vi "Dynamic Launch Nested Actor.vi"(8 "error in (no error)":errorcluster, 11 "UI ActorTop in":refnum<class "UI_Top.lvclass">) -> (0 "error out":errorcluster, 3 "UI ActorTop out":refnum<class "UI_Top.lvclass">)   [LabVIEW 2021, in "UI_Top.lvclass"]
doc: "Use Launch Nested Actor.vi to dynamic load child VI.\n2015-04-02 12:54:56\n蒋松\njiangsong@outlook.com"
uses:
  UI_Top.lvclass
  C:/Program Files (x86)/National Instruments/LabVIEW 2021/vi.lib/ActorFramework/Actor/Actor.lvclass
  C:/Program Files (x86)/National Instruments/LabVIEW 2021/user.lib/John_Lib/AbstractActorTemplate/AbstractActorTemplate/UIActorTop.lvclass
  UI_Top.lvclass/UI_Top.ctl
  <vilib>/ActorFramework/Actor/Actor.lvclass
  C:/Program Files (x86)/National Instruments/LabVIEW 2021/project/Create Actor from Template/Source_DataViewer/UI_Top/UI_Top.lvclass
  C:/Program Files (x86)/National Instruments/LabVIEW 2021/user.lib/John_Lib/Interfaces/InsertMainSubPanel/InsertMainSubPanel.lvclass
  C:/Program Files (x86)/National Instruments/LabVIEW 2021/user.lib/John_Lib/Interfaces/Windows Title/Windows Title.lvclass
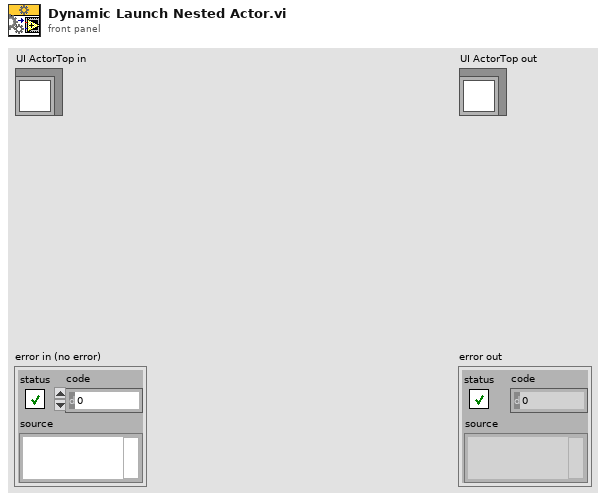
[diagram p1: front panel]
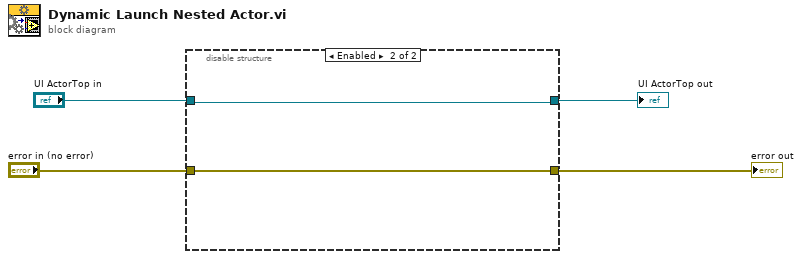
[diagram p0: block diagram]
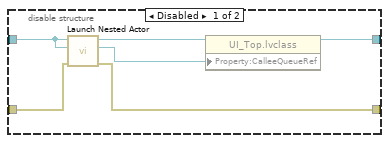
[diagram p2: hidden frame]
diagram:
  n1 = disable-structure shown="Enabled" {
    disable-tunnel: "error in (no error)" -> [w9 w11]
    disable-tunnel: [w8 w11] -> w3
    disable-tunnel: [w7 w12] -> w2
    disable-tunnel: "UI ActorTop in" -> [w5 w12]
    frame Disabled {
      n2 = call <vilib>:"Launch Nested Actor.vi"("error in (no error)"=w9, "Nested Actor"=w5, "Caller Actor in"=w5) -> ("error out"=w8:errorcluster, "Nested Actor's Enqueuer"=w6:refnum<class "Message Enqueuer.lvclass">, "Caller Actor out"=w10:refnum<class "UI_Top.lvclass">)  [unwired: 6 in]
      n3 = property class="UI_Top.lvclass"(reference=w10, "Property:CalleeQueueRef"=w6) -> (reference out=w7:refnum<class "UI_Top.lvclass">)  [unwired: 1 in, 1 out]
    }
    frame Enabled {
    }
  }
  "error out" <- w3
  "UI ActorTop out" <- w2
